vi "ReadRecord.vi"(8 "error in":errorcluster, 11 "scope params":T1={"scope mode"=enum."Stopped", "ticker"=refnum, "samples per simulated"=0, "FPGA ref"=refnum, "P2P params"={"instrument handle"="", "stream session"=refnum, "scale"={"offset"=0.0, "gain"=0.0, "reserved 1"=0.0, "reserved 2"=0.0}, "actual sample rate"=10000000.0, "Trigger"=enum."PFI 0", "SCOPE Resource"="Dev1", "input impedance"=0}, "data mode"=enum."Real IO"} {"P2P params"."input impedance" items=["1 mega ohm"=0, "50 ohms"=2]; "P2P params"."actual sample rate" format="%.2p"}) -> (0 "error out":errorcluster, 2 "data":dbl[][](array[numeric]) format="%.2f", 3 "scope params out":T1={"scope mode"=enum."Stopped", "ticker"=refnum, "samples per simulated"=0, "FPGA ref"=refnum, "P2P params"={"instrument handle"="", "stream session"=refnum, "scale"={"offset"=0.0, "gain"=0.0, "reserved 1"=0.0, "reserved 2"=0.0}, "actual sample rate"=10000000.0, "Trigger"=enum."PFI 0", "SCOPE Resource"="Dev1", "input impedance"=0}, "data mode"=enum."Real IO"} {"P2P params"."input impedance" items=["1 mega ohm"=0, "50 ohms"=2]; "P2P params"."actual sample rate" format="%.2p"})   [LabVIEW 2013]
uses:
  <vilib>/rvi/interface/nirviReadWriteControl/nirviReadWriteControl.xnode
  NiFpgaLv.dll
  <vilib>/Utility/error.llb/Error Cluster From Error Code.vi
  <vilib>/rvi/interface/Simulation/niFpgaSimulationCallBeginRW.vi
  <vilib>/rvi/errors/niLvFpgaAdjustHostInterfaceError.vi
  <vilib>/rvi/interface/nirviMethod/nirviMethod.xnode
  Config/FPGAref.ctl
  <vilib>/FPGAPlugInAG/Dynamic/niLvFpga_ReadFifo_Dynamic.vi
  <vilib>/rvi/errors/niLvFpgaMergeErrorWithErrorCode.vi
  controls/ScopeMode.ctl
  Utilities/Ticker/Ticker.lvclass
  controls/scope_params.ctl
  P2P streaming/P2P params.ctl
  P2P streaming/trigger_source.ctl
  FPGA/DataMode.ctl
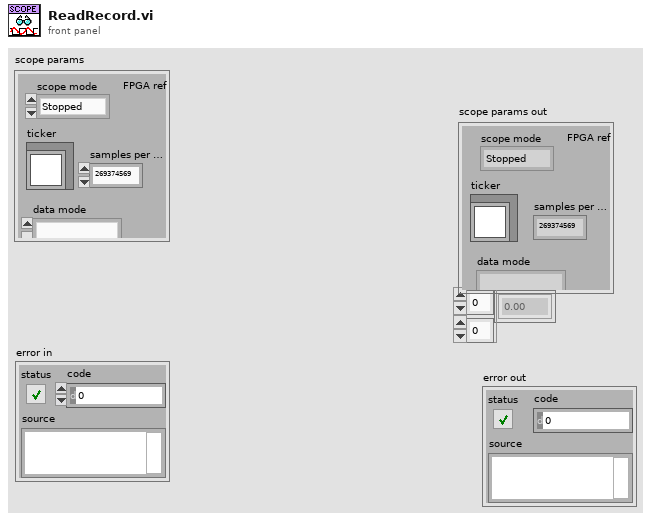
[diagram p1: front panel]
types:
  T1 = typedef "scope_params.ctl" = cluster{"scope mode":T2, "ticker":refnum<class "Ticker.lvclass">, "samples per simulated":u32, "FPGA ref":T3, "P2P params":T4, "data mode":T6}
  T2 = typedef "ScopeMode.ctl" = enum16{"Stopped", "Single", "Running"}
  T3 = typedef "FPGAref.ctl" = refnum<k20>
  T4 = typedef "P2P params.ctl" = cluster{"instrument handle":refnum<k15>, "stream session":refnum<k20>, "scale":cluster{"offset":dbl, "gain":dbl, "reserved 1":dbl, "reserved 2":dbl}, "actual sample rate":dbl, "Trigger":T5, "SCOPE Resource":refnum<k15>, "input impedance":u32}
  T5 = typedef "trigger_source.ctl" = enum16{"PFI 0", "PFI 1", "Software"}
  T6 = typedef "DataMode.ctl" = enum16{"Real IO", "Simulated"}
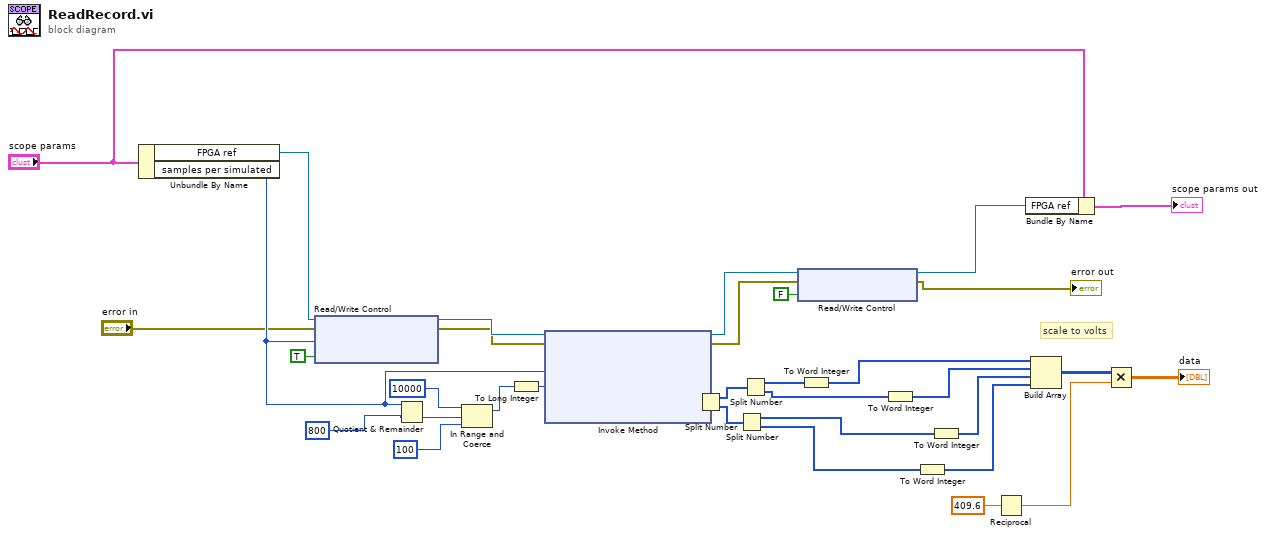
[diagram p0: block diagram]
diagram:
  # "scale to volts"
  n1 = Unbundle By Name("scope params") -> ("FPGA ref"=w8:T3, "samples per simulated"=w15:u32)
  n2 = xnode "Read/Write Control"("FPGA VI Reference In"=w8, "error in"="error in", "Samples Per Trigger"=w15, "Trigger Acquisition"=TRUE) -> ("FPGA VI Reference Out"=w33:T3, "error out"=w18:errorcluster)
  n3 = Quotient & Remainder(x=w15, y=u32 800) -> (floor(x/y)=w22:u32)  [unwired: 1 out]
  n4 = In Range and Coerce(upper limit=u32 10000, x=w22, lower limit=u32 100) -> (coerced(x)=w19:u32)  [unwired: 1 out]
  n5 = To Long Integer(number=w19) -> (32bit integer=w14:i32)
  n6 = xnode "Invoke Method"("FPGA VI Reference In"=w33, "error in"=w18, "Number of Elements"=w15, "Timeout (ms)"=w14) -> ("FPGA VI Reference Out"=w24:T3, "error out"=w17:errorcluster, "Data"=w30:u64[])  [unwired: 1 out]
  n7 = Split Number(x=w30) -> (hi(x)=w32:u32[], lo(x)=w31:u32[])
  n8 = Split Number(x=w31) -> (hi(x)=w28:u16[], lo(x)=w27:u16[])
  n9 = Split Number(x=w32) -> (hi(x)=w26:u16[], lo(x)=w29:u16[])
  n10 = xnode "Read/Write Control"("FPGA VI Reference In"=w24, "error in"=w17, "Trigger Acquisition"=FALSE) -> ("FPGA VI Reference Out"=w6:T3, "error out"=→"error out":errorcluster)
  n11 = To Word Integer(number=w26) -> (16bit integer=w13:i16[])
  n12 = To Word Integer(number=w29) -> (16bit integer=w12:i16[])
  n13 = To Word Integer(number=w27) -> (16bit integer=w10:i16[])
  n14 = To Word Integer(number=w28) -> (16bit integer=w11:i16[])
  n15 = Reciprocal(x=409.6) -> (1/x=w3:dbl)
  n16 = Bundle By Name(cluster="scope params", "FPGA ref"=w6) -> (→"scope params out":T1)
  n17 = Build Array(w13, w12, w11, w10) -> (w2:i16[][])
  n18 = Multiply(x=w2, y=w3) -> (x*y=→"data":dbl[][])
